vi "Camera_EdgHorzObjThreshold.vi"(8 "error in (no error)":errorcluster, 10 "Threshold":i8(slide)=4 scale=1.0..9.0, 11 "SRV In":refnum<k5>) -> (0 "error out":errorcluster, 3 "SRV Out":refnum<k5>)   [LabVIEW 2014]
doc: "Sets the camera threshold.\n\n\nModified for Benilde St. Margaret's School - Tim Jump\nBy Doug Schmertman - Logic PD\nCopyright 2012"
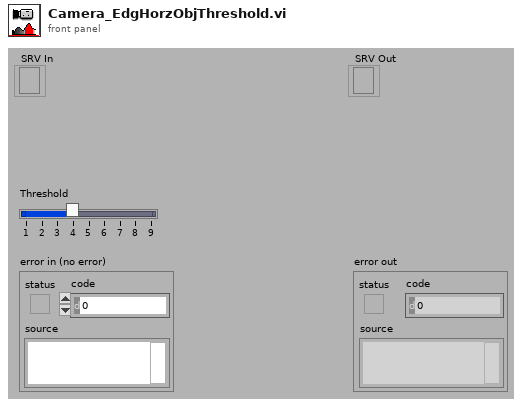
[diagram p1: front panel]
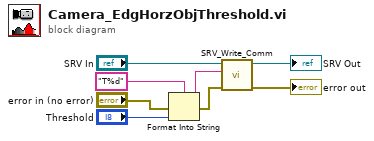
[diagram p0: block diagram]
diagram:
  n1 = Format Into String(format string="T%d" ("Command Sent"), error in="error in (no error)", "Threshold") -> (resulting string=w5:string, error out=w4:errorcluster)  [unwired: 1 in]
  n2 = call "SRV_Write_Comm.vi"("error in (no error)"=w4, "Command Sent"=w5, "SRV In"="SRV In") -> ("error out"=→"error out":errorcluster, "SRV Out"=→"SRV Out":refnum<k5>)  [unwired: 6 in, 1 out]
